vi "DisconnectRobot.vi"(0 "Universal Robot.lvclass in":refnum<class "Universal Robot.lvclass">, 5 "error in (no error)":errorcluster) -> (14 "Universal Robot.lvclass out":refnum<class "Universal Robot.lvclass">, 19 "error out":errorcluster)   [LabVIEW 2019, in "Universal Robot.lvclass"]
uses:
  Universal Robot.lvclass
  Universal Robot.lvclass/Universal Robot.ctl
  Client Interfaces/Dashboard Server/Dashboard Server.lvclass
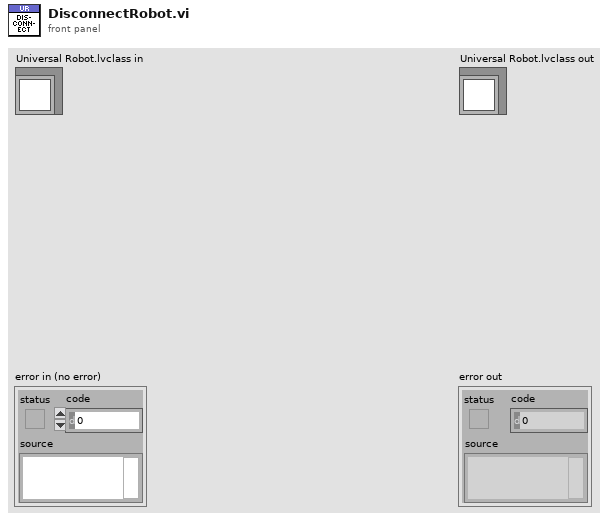
[diagram p1: front panel]
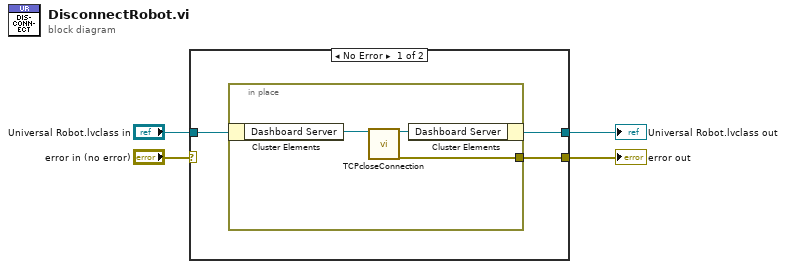
[diagram p0: block diagram]
diagram:
  n1 = case shown="No Error" "error in (no error)" {
    selector: "error in (no error)" -> [_ w12]
    tunnel: [w6 w12] -> w3
    tunnel: "Universal Robot.lvclass in" -> [w7 w11]
    tunnel: [w5 w11] -> w1
    frame No Error {
      n2 = in-place {
        in-place-border: [w8] -> w6
        n3 = in-place-cluster #1(w7) -> ("Dashboard Server"=w10:refnum<class "Dashboard Server.lvclass">)
        n4 = call-dynamic "TCPcloseConnection.vi"("DashboardServer in"=w10) -> ("DashboardServer out"=w9:refnum<class "Dashboard Server.lvclass">, "error out"=w8:errorcluster)  [unwired: 17 in]
        n5 = in-place-cluster #1("Dashboard Server"=w9) -> (w5:refnum<class "Universal Robot.lvclass">)
      }
    }
    frame Error {
    }
  }
  "error out" <- w3
  "Universal Robot.lvclass out" <- w1
